vi "Start_Client.vi"(7 "Run exec":bool, 8 "error in":errorcluster, 9 "Module Name":string="az_exec_200218.vi", 10 "Alarms in":T1, 11 "VI in":refnum<vi>) -> (0 "error out":errorcluster, 1 "running":bool, 2 "Execution:State":T4(ring), 3 "VI out":refnum<vi>)   [LabVIEW 2019]
uses:
  Alarms/Ctl/Alarms.ctl
  Alarms/Ctl/ALR_defs.ctl
  Alarms/Ctl/ALRs_State.ctl
  Alarms/Ctl/ALR_ON_OFF.ctl
  Alarms/Ctl/ALR_Parameters.ctl
  Alarms/Ctl/ALR code.ctl
  Alarms/Ctl/ALR type.ctl
  Logik/Logik.lvlib
  Alarms/Alarms.lvlib
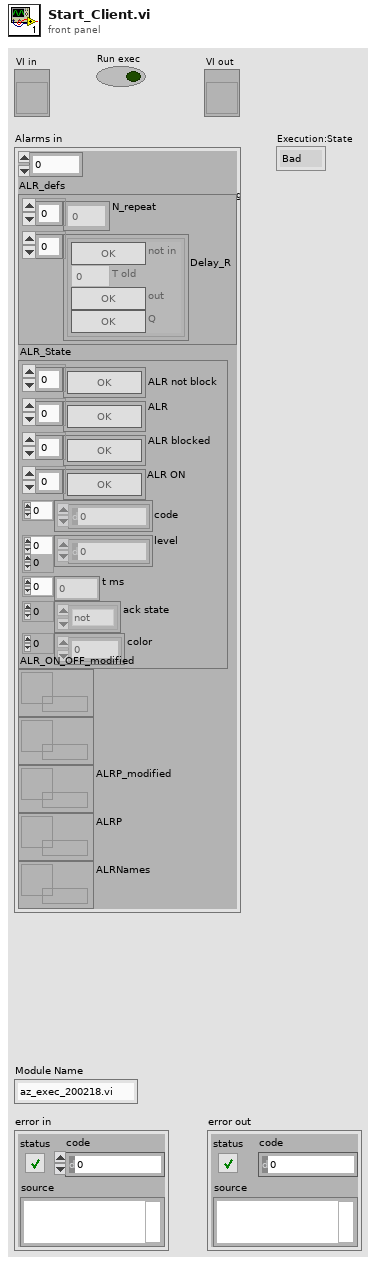
[diagram p1: front panel]
types:
  T1 = typedef "Alarms.lvlib/Alarms.ctl" = cluster{"N_param":i32, "ALR_defs":T2, "ALR_State":T3, "ALR_ON_OFF_modified":refnum<data-value>, "ALR_ON_OFF":refnum<data-value>, "ALRP_modified":refnum<data-value>, "ALRP":refnum<data-value>, "ALRNames":refnum<data-value>}
  T2 = typedef "Alarms.lvlib/ALR_defs.ctl" = cluster{"N_repeat":u32[], "Delay_R":cluster{"not in":bool, "T old":u32, "out":bool, "Q":bool}[]}
  T3 = typedef "Alarms.lvlib/ALRs_State.ctl" = cluster{"ALR not block":bool[], "ALR":bool[], "ALR blocked":bool[], "ALR ON":bool[], "code":i32[], "level":i32[][], "t ms":u32[], "ack state":enum32{"not", "tripped", "reset", "ack"}[], "color":u32[]}
  T4 = enum32{"Bad", "Idle", "Run top level", "Running"}
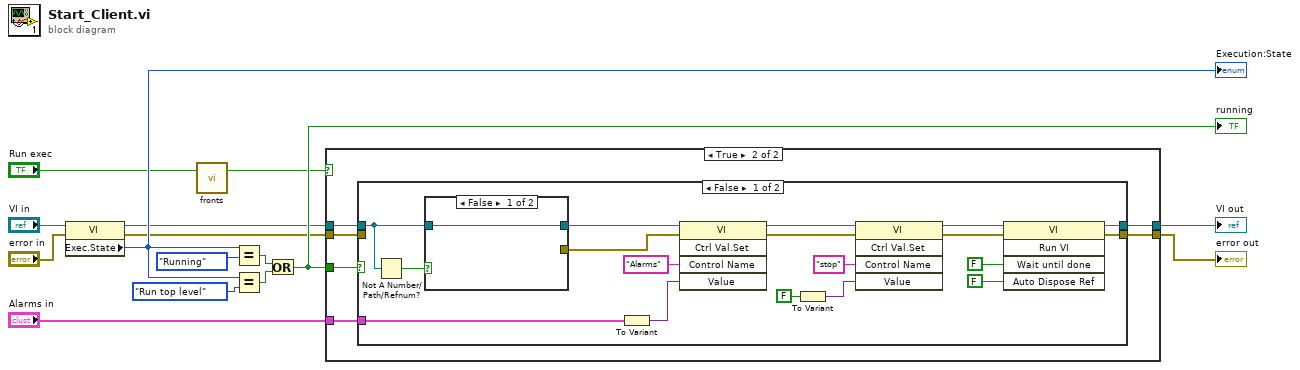
[diagram p0: block diagram]
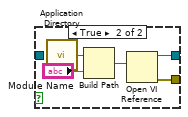
[diagram p3: hidden frame]
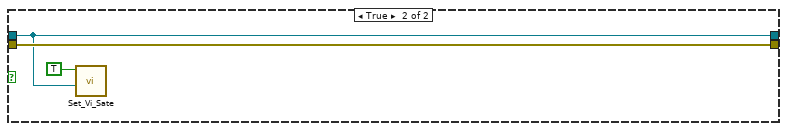
[diagram p4: hidden frame]
diagram:
  n1 = property class="VI"(reference="VI in", error in="error in") -> (reference out=w9:refnum<vi>, error out=w10:errorcluster, "Exec.State"=w13:T4)
  "Execution:State" <- w13
  n2 = call "fronts.vi"("in"="Run exec") -> ("raise"=w2:bool)  [unwired: 1 in, 1 out]
  n3 = Equal?(x=w13, y=T4."Running") -> (x = y?=w11:bool)
  n4 = Equal?(x=w13, y=T4."Run top level") -> (x = y?=w15:bool)
  n5 = Or(x=w11, y=w15) -> (x .or. y?=w14:bool)
  "running" <- w14
  n6 = case shown="True" w2 {
    tunnel: "Alarms in" -> [_ w23]
    tunnel: [w17 w22] -> w5
    tunnel: [w16 w21] -> w6
    tunnel: w9 -> [w17 w20]
    tunnel: w10 -> [w16 w19]
    tunnel: w14 -> [_ w18]
    frame False {
    }
    frame True {
      n7 = case shown="False" w18 {
        tunnel: w23 -> [w35 _]
        tunnel: [w34 w48] -> w22
        tunnel: [w33 w49] -> w21
        tunnel: w20 -> [w24 w48]
        tunnel: w19 -> [_ w49]
        frame False {
          n8 = Not A Number/Path/Refnum?(number/path/refnum=w24) -> (NaN/Path/Refnum?=w25:bool)
          n9 = case shown="False" w25 {
            tunnel: [w42 w47] -> w41
            tunnel: [_ w46] -> w40
            tunnel: w24 -> [w42 _]
            frame False {
            }
            frame True {
              n10 = call <vilib>:"Application Directory.vi"() -> ("Application Directory"=w43:path)
              n11 = Build Path(base path=w43, name or relative path="Module Name") -> (appended path=w44:path)
              n12 = Open VI Reference(vi path=w44) -> (vi reference=w47:refnum<vi>, error out=w46:errorcluster)  [unwired: 5 in]
            }
          }
          n13 = To Variant(anything=w35) -> (Variant=w39:variant)
          n14 = invoke class="VI" method="Ctrl Val.Set"(reference=w41, error in=w40, "Control Name"="Alarms", "Value"=w39) -> (reference out=w29:refnum<vi>, error out=w28:errorcluster)  [unwired: 1 in, 3 out]
          n15 = To Variant(anything=FALSE ("Auto Dispose Ref")) -> (Variant=w31:variant)
          n16 = invoke class="VI" method="Ctrl Val.Set"(reference=w29, error in=w28, "Control Name"="stop", "Value"=w31) -> (reference out=w27:refnum<vi>, error out=w26:errorcluster)  [unwired: 1 in, 3 out]
          n17 = invoke class="VI" method="Run VI"(reference=w27, error in=w26, "Wait until done"=FALSE, "Auto Dispose Ref"=FALSE) -> (reference out=w34:refnum<vi>, error out=w33:errorcluster)  [unwired: 1 in, 3 out]
        }
        frame True {
          n18 = call "Set_Vi_Sate.vi"("VI"=w48, "Activate (F)"=TRUE) -> ()  [unwired: 9 in, 1 out]
        }
      }
    }
  }
  "error out" <- w6
  "VI out" <- w5
